vi "JogAxis.vi"(8 "error in (no error)":errorcluster, 9 "Steps":i32, 10 "Axis":T1, 11 "MotorController in":refnum<class "MotorController.lvclass">) -> (0 "error out":errorcluster, 3 "MotorController out":refnum<class "MotorController.lvclass">)   [LabVIEW 2019, in "MotorController.lvclass"]
uses:
  MotorController.lvclass
  Axes_enum_typedef.ctl
  MotorController.lvclass/MotorController.ctl
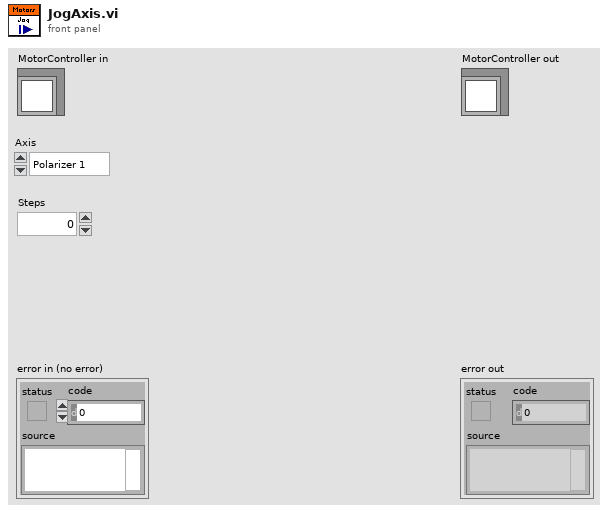
[diagram p1: front panel]
types:
  T1 = typedef "Axes_enum_typedef.ctl" = enum16{"Polarizer 1", "Polarizer 2", "Sample", "Stage"}
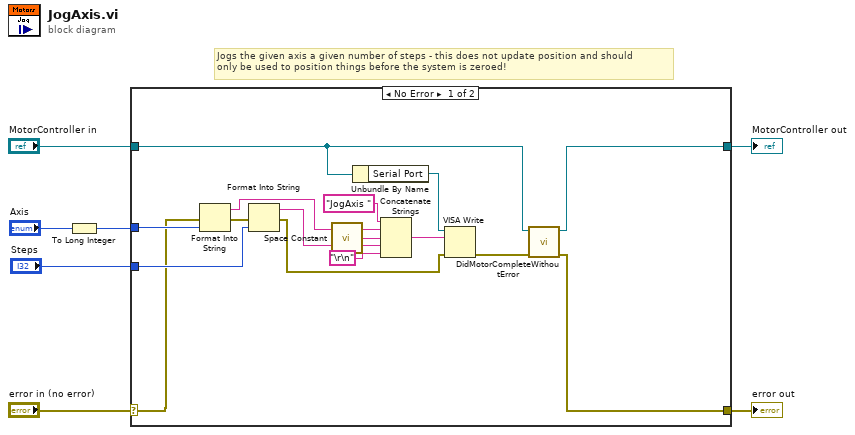
[diagram p0: block diagram]
diagram:
  # "Jogs the given axis a given number of steps - this does not update position and should\nonly be used to position things before the system is zeroed!"
  n1 = To Long Integer(number="Axis") -> (32bit integer=w2:i32)
  n2 = case shown="No Error" "error in (no error)" {
    selector: "error in (no error)" -> [w20 w25]
    tunnel: [w10 w25] -> w6
    tunnel: [w8 w24] -> w4
    tunnel: "MotorController in" -> [w9 w24]
    tunnel: w2 -> [w23 _]
    tunnel: "Steps" -> [w21 _]
    frame No Error {
      n3 = Format Into String(error in=w20, w23) -> (resulting string=w18:string, error out=w22:errorcluster)  [unwired: 2 in]
      n4 = Format Into String(error in=w22, w21) -> (resulting string=w17:string, error out=w12:errorcluster)  [unwired: 2 in]
      n5 = call <vilib>:"Space Constant.vi"() -> ("String"=w16:string)
      n6 = Unbundle By Name(w9) -> ("Serial Port"=w14:refnum<visa-resource-name>)
      n7 = Concatenate Strings("JogAxis ", w18, w16, w17, "\r\n") -> (w13:string)
      n8 = VISA Write(VISA resource name=w14, write buffer=w13, error in (no error)=w12) -> (error out=w11:errorcluster)  [unwired: 2 out]
      n9 = call "DidMotorCompleteWithoutError.vi"("error in (no error)"=w11, "MotorController in"=w9) -> ("error out"=w10:errorcluster, "MotorController out"=w8:refnum<class "MotorController.lvclass">)  [unwired: 7 in, 1 out]
    }
    frame Error {
    }
  }
  "error out" <- w6
  "MotorController out" <- w4
